vi "LogExpiredProcess.vi"(8 "error in":errorcluster, 10 "Expired Process":string, 11 "Path":path) -> (0 "error out":errorcluster)   [LabVIEW 2017, in "WatchdogProcess.lvlib"]
doc: "Specifies the length of the hardware timeout period that triggers a recovery procedure."
uses:
  <vilib>/addons/WatchdogProcess/WatchdogProcess.lvlib
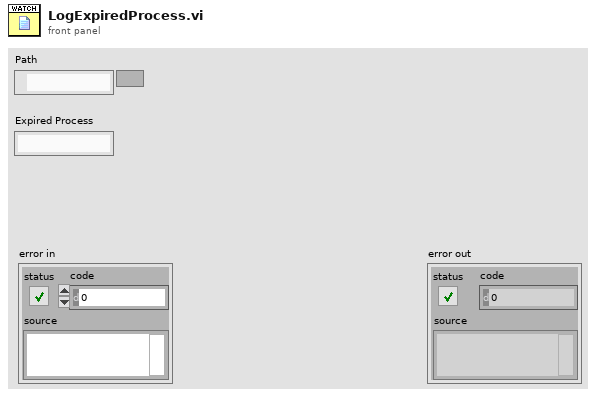
[diagram p1: front panel]
types:
  T1 = enum16{"open", "replace", "create", "open or create", "replace or create", "replace or create with confirmation"}
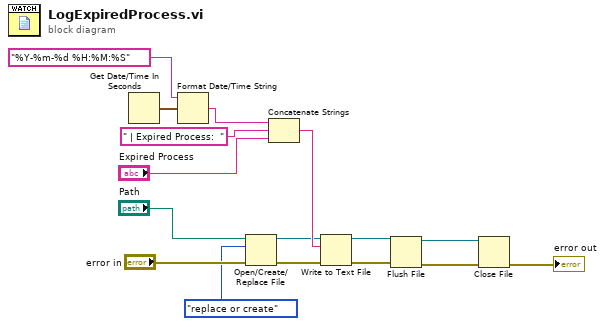
[diagram p0: block diagram]
diagram:
  n1 = Get Date/Time In Seconds() -> (seconds since 1Jan1904=w13:timestamp)
  n2 = Format Date/Time String(time format string (%c)="%Y-%m-%d %H:%M:%S", seconds (now)=w13) -> (date/time string=w11:string)  [unwired: 1 in]
  n3 = Open/Create/Replace File(file path (use dialog)="Path", error in="error in", operation (0:open)=T1."replace or create") -> (refnum out=w7:refnum<file>, error out=w6:errorcluster)  [unwired: 3 in, 1 out]
  n4 = Concatenate Strings(w11, " | Expired Process:  " ("string"), "Expired Process") -> (w8:string)
  n5 = Write to Text File(file (use dialog)=w7, text=w8, error in=w6) -> (refnum out=w5:refnum<file>, error out=w4:errorcluster)  [unwired: 1 in, 1 out]
  n6 = Flush File(refnum=w5, error in=w4) -> (refnum out=w3:refnum<file>, error out=w2:errorcluster)
  n7 = Close File(refnum=w3, error in=w2) -> (error out=→"error out":errorcluster)  [unwired: 1 out]
